vi "Publish message (SubVI).vi"(0 "Exchange in":refnum<class "Exchange.lvclass">, 1 "target":string, 2 "body":u8[](array[numeric]), 3 "error in (no error)":errorcluster, 4 "MessageProperties":refnum<k24>) -> (5 "Exchange out":refnum<class "Exchange.lvclass">, 7 "error out":errorcluster)   [LabVIEW 2016]
uses:
  <vilib>/Distrio/LabbitMQ/Exchange/Exchange.lvclass
  C:/Program Files (x86)/National Instruments/LabVIEW 2016/vi.lib/Distrio/LabbitMQ/RabbitMQ.Client.dll
  Program Files (x86)/National Instruments/LabVIEW 2016/vi.lib/Distrio/LabbitMQ/RabbitMQ.Client.dll
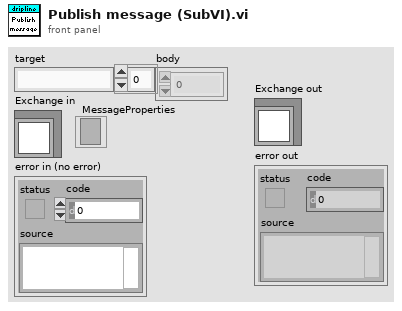
[diagram p1: front panel]
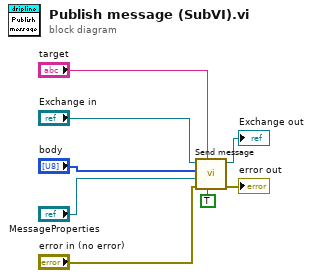
[diagram p0: block diagram]
diagram:
  n1 = call <vilib>:"Send message.vi"("mandatory? (F)"=TRUE, "routing key"="target", "error in (no error)"="error in (no error)", "MessageProperties"="MessageProperties", "body"="body", "Exchange in"="Exchange in") -> ("error out"=→"error out":errorcluster, "Exchange out"=→"Exchange out":refnum<class "Exchange.lvclass">)  [unwired: 4 in]
